vi "ValidateScan.vi"(8 "error in (no error)":errorcluster, 9 "LF?":bool, 11 "String In":string) -> (0 "error out":errorcluster, 1 "Valid Format?":bool, 2 "ScanData":T1, 3 "String Out":string)   [LabVIEW 2015]
uses:
  Controls/Scanned Data.ctl
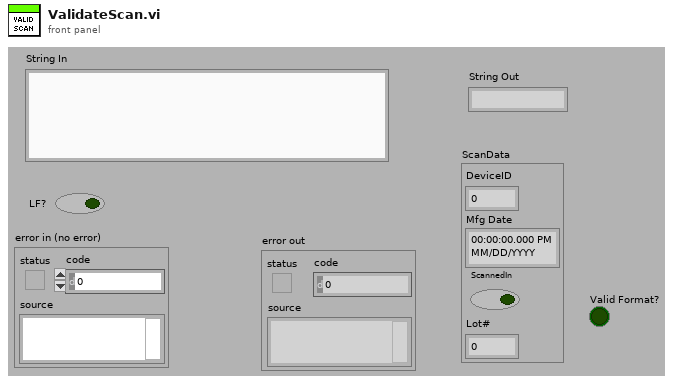
[diagram p1: front panel]
types:
  T1 = typedef "Scanned Data.ctl" = cluster{"DeviceID":u32, "Mfg Date":timestamp, "ScannedIn":bool, "Lot#":u32}
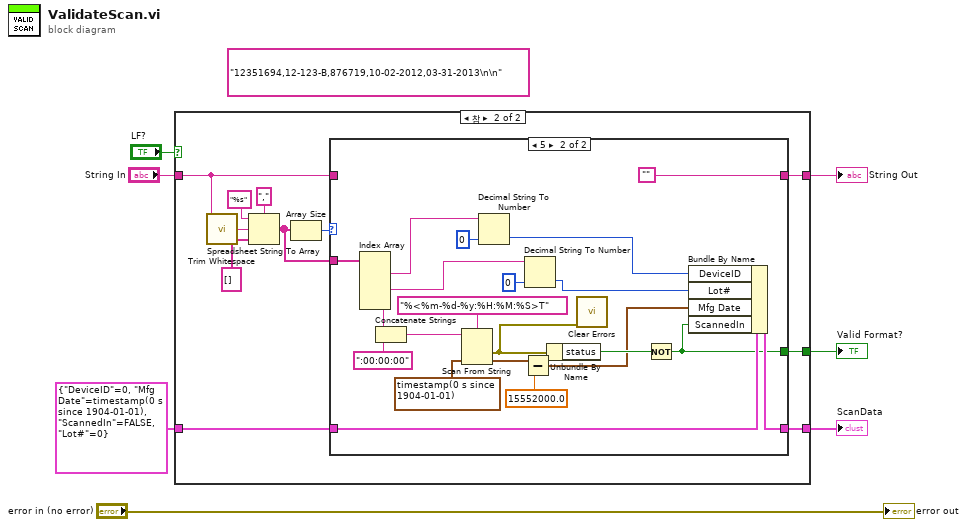
[diagram p0: block diagram]
diagram:
  (unwired) "12351694,12-123-B,876719,10-02-2012,03-31-2013\n\n"
  n1 = case shown="참" "LF?" {
    tunnel: [w9 w20] -> w7
    tunnel: T1 {"DeviceID"=0, "Mfg Date"=timestamp(0 s since 1904-01-01), "ScannedIn"=FALSE, "Lot#"=0} ("Cluster") -> [w8 w19]
    tunnel: [w8 w18] -> w3
    tunnel: [_ w17] -> w4
    tunnel: "String In" -> [w9 w16]
    frame False {
    }
    frame True {
      n2 = call <vilib>:"Trim Whitespace.vi"("string"=w16) -> ("trimmed string"=w12:string)  [unwired: 1 in]
      n3 = Spreadsheet String To Array(delimiter (Tab)=",", format string="%s", spreadsheet string=w12, array type (2D Dbl)=string[] []) -> (array=w10:string[])
      n4 = Array Size(array=w10) -> (size(s)=w11:i32)
      n5 = case shown="5" w11 {
        tunnel: [w21 ""] -> w20
        tunnel: w19 -> [w22 w42]
        tunnel: [w22 w41] -> w18
        tunnel: [_ w29] -> w17
        tunnel: w16 -> [w21 _]
        tunnel: w10 -> [_ w40]
        frame Default {
        }
        frame 5 {
          n6 = Index Array(array=w40) -> (element #1=w28:string, element #3=w25:string, element #5=w35:string)  [unwired: 5 in, 2 out]
          n7 = Concatenate Strings(w35, ":00:00:00" ("string")) -> (w38:string)
          n8 = Scan From String(format string="%<%m-%d-%y:%H:%M:%S>T", input string=w38, default 1=timestamp(0 s since 1904-01-01) ("current time")) -> (error out=w32:errorcluster, output 1=w34:timestamp)  [unwired: 2 in, 2 out]
          n9 = Decimal String To Number(string=w28, default (0L)=u32 0 ("default (0 I32)")) -> (number=w26:u32)  [unwired: 1 in, 1 out]
          n10 = Subtract(x=w34, y=15552000.0) -> (x-y=w30:timestamp)
          n11 = Decimal String To Number(string=w25, default (0L)=u32 0 ("default (0 I32)")) -> (number=w24:u32)  [unwired: 1 in, 1 out]
          n12 = Unbundle By Name(w32) -> ("status"=w31:bool)
          n13 = call <vilib>:"Clear Errors.vi"("error in (no error)"=w32) -> ()  [unwired: 5 in, 2 out]
          n14 = Not(x=w31) -> (.not. x?=w29:bool)
          n15 = Bundle By Name(cluster=w42, "DeviceID"=w26, "Lot#"=w24, "Mfg Date"=w30, "ScannedIn"=w29) -> (w41:T1)
        }
      }
    }
  }
  "String Out" <- w7
  "Valid Format?" <- w4
  "ScanData" <- w3
  "error out" <- "error in (no error)"
